vi "flot graph for  year.vi"(7 "BD Date":string[](array[string]), 8 "error in (no error)":errorcluster, 10 "number":dbl[](array[numeric]), 11 "Count total":string[](array[string])) -> (0 "error out":errorcluster, 3 "Run-Time Status":cluster{"Array 2":timestamp[], dbl[]}(graph))   [LabVIEW 2017]
panel:
  out "element":timestamp
  out "Elements Found out 2":string[](array[string])
  in  "1":dbl format="%#_13g"
  out "XY Graph":cluster{"Array 2":timestamp[], dbl[]}(graph)
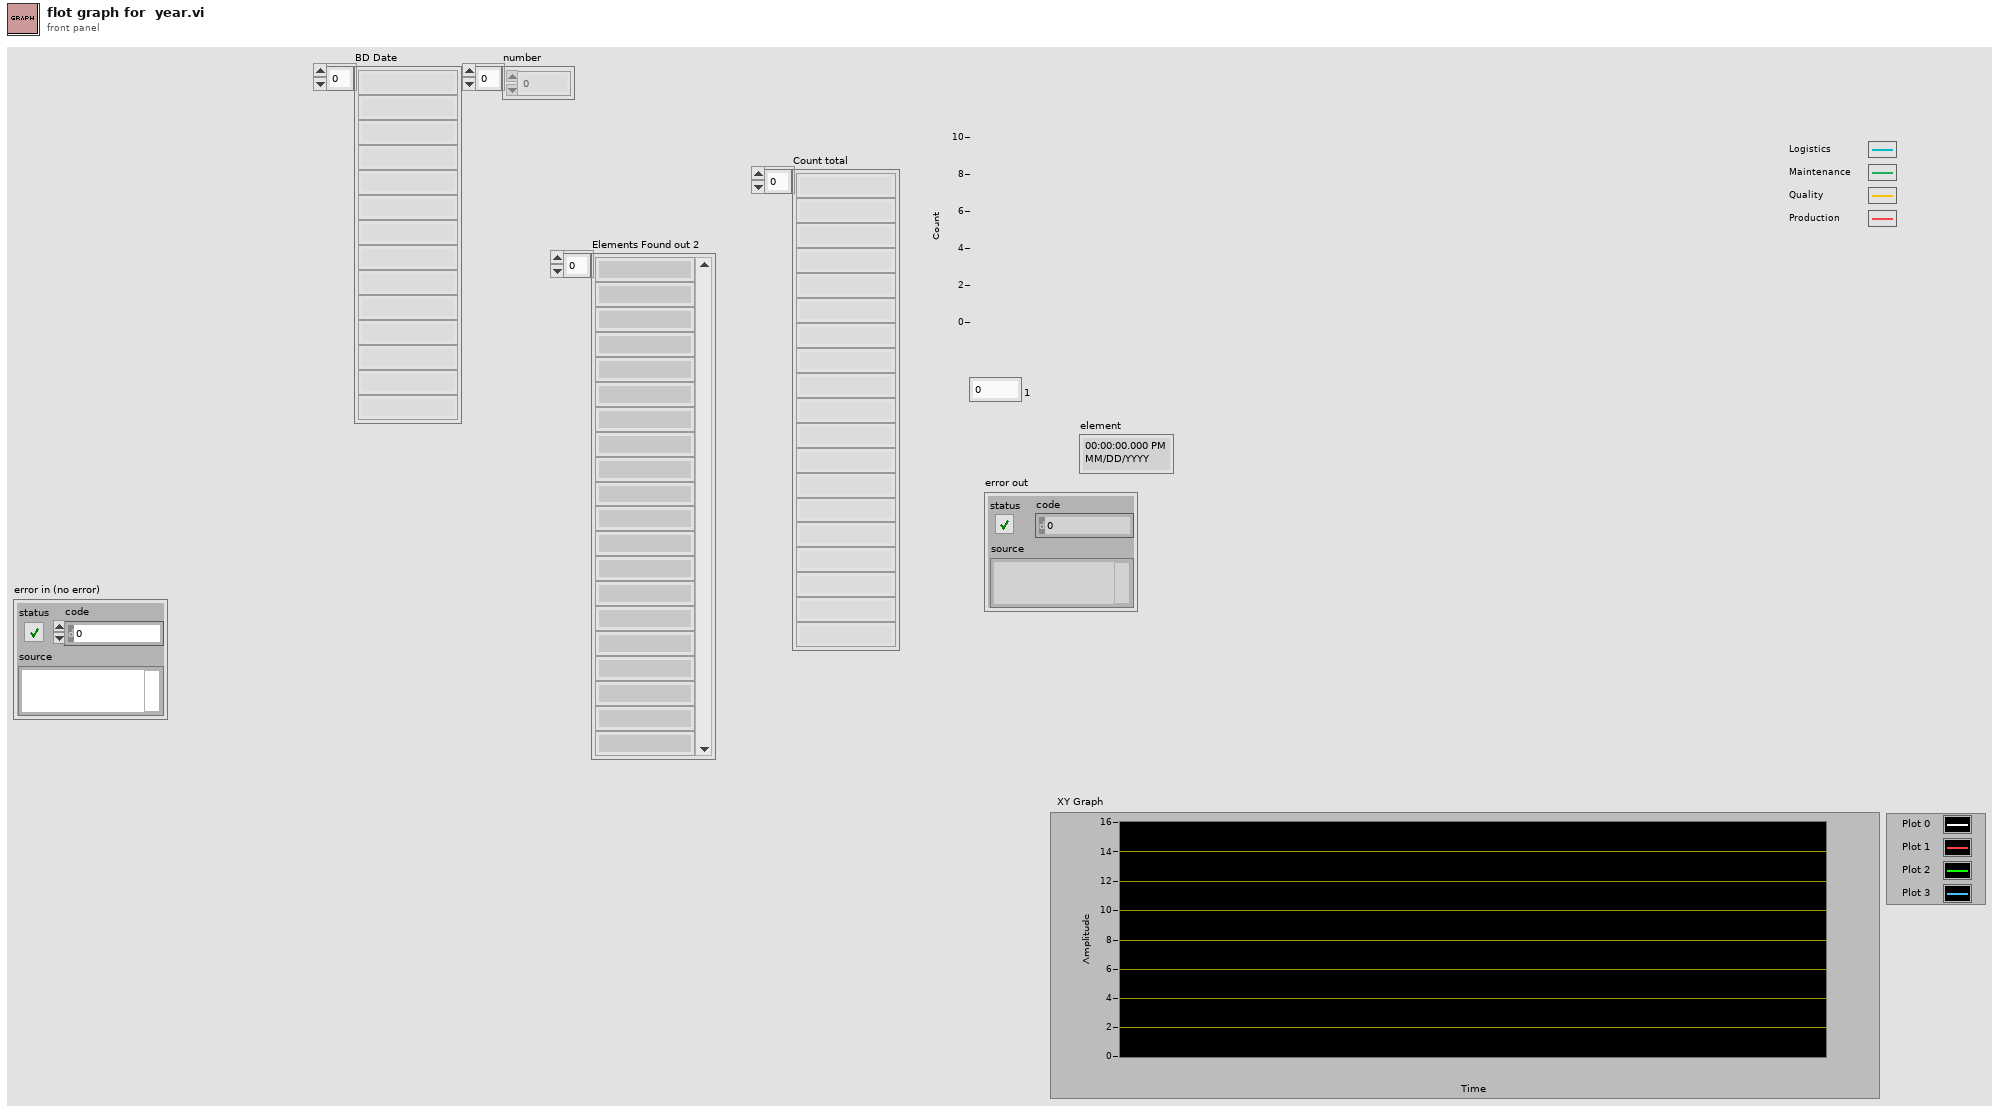
[diagram p1: front panel]
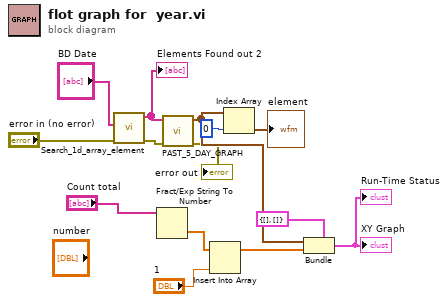
[diagram p0: block diagram]
diagram:
  n1 = call "Search_1d_array_element.vi"("error in (no error)"="error in (no error)", "BD Date"="BD Date") -> ("error out"=w3:errorcluster, "Elements Found out"=w7:string[])  [unwired: 5 in, 1 out]
  "Elements Found out 2" <- w7
  n2 = Fract/Exp String To Number(string="Count total") -> (number=w1:dbl[])  [unwired: 3 in, 1 out]
  n3 = call "PAST_5_DAY_GRAPH.vi"("error in (no error) 2"=w3, "5 date"=w7) -> ("error out"=→"error out":errorcluster, "Array 2"=w11:timestamp[])  [unwired: 8 in]
  n4 = Insert Into Array(array=w1, new element="1") -> (w13:dbl[])  [unwired: 1 in]
  n5 = Index Array(array=w11, index=0) -> (element=→"element":timestamp)
  n6 = Bundle(cluster=cluster{"Array 2":timestamp[], dbl[]} {"Array 2"=[], []}, "Array 2"=w11, w13) -> (→"XY Graph" →"Run-Time Status":cluster{"Array 2":timestamp[], dbl[]})
